vi "STFT Calculation.vi"(1 "time increment":i32, 2 "g":dbl[](array[numeric]) format="%.2f", 3 "s":dbl[](array[numeric]) format="%.2f") -> (0 "Fourier[s(i-m)*g(m)]":dbl[][](array[numeric]) format="%.2f")   [LabVIEW 2017, in "NI_Gmath.lvlib"]
uses:
  <vilib>/gmath/NI_Gmath.lvlib
  <vilib>/Analysis/2dsp.llb/Real FFT.vi
  <vilib>/Analysis/NI_AALPro.lvlib
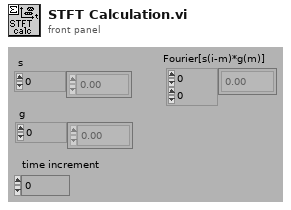
[diagram p1: front panel]
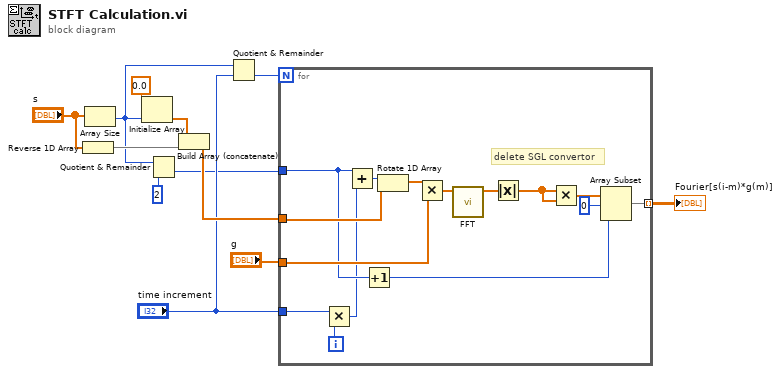
[diagram p0: block diagram]
diagram:
  n1 = Reverse 1D Array(array="s") -> (reversed array=w11:dbl[])
  n2 = Array Size(array="s") -> (size(s)=w3:i32)
  n3 = Initialize Array(sgl 0.0, w3) -> (w10:sgl[])
  n4 = Quotient & Remainder(x=w3, y=2) -> (floor(x/y)=w4:i32)  [unwired: 1 out]
  n5 = Build Array (concatenate)(w10, w11) -> (w7:dbl[])
  n6 = Quotient & Remainder(x=w3, y="time increment") -> (floor(x/y)=w2:i32)  [unwired: 1 out]
  n7 = for {
    N: w2 -> [_]
    tunnel: "g" -> [w27]
    tunnel: w7 -> [w26]
    tunnel: "time increment" -> [w23]
    tunnel: w4 -> [w25]
    tunnel: [w21] -> w1 mode=indexing
    i -> [w24]
    # "delete SGL convertor"
    n8 = Multiply(x=w23, y=w24) -> (x*y=w22:i32)
    n9 = Add(x=w25, y=w22) -> (x+y=w20:i32)
    n10 = Increment(x=w25) -> (x+1=w17:i32)
    n11 = Rotate 1D Array(1:w26, 2:w20) -> (0:w19:dbl[])
    n12 = Multiply(x=w19, y=w27) -> (x*y=w16:dbl[])
    n13 = call-poly <vilib>:"FFT.vi"("X"=w16) -> ("FFT {X}"=w15:cdb[])  [unwired: 9 in, 1 out]
    n14 = Absolute Value(x=w15) -> (abs(x)=w13:dbl[])
    n15 = Multiply(x=w13, y=w13) -> (x*y=w14:dbl[])
    n16 = Array Subset(array=w14, index=0, length=w17) -> (w21:dbl[])
  }
  "Fourier[s(i-m)*g(m)]" <- w1
